vi "DAQmx_Express_mod.vi"(2 "rate":dbl=0.3, 3 "number of samples":i32=1, 4 "timeout (s)":dbl=10.0 format="%0.2f", 5 "error in":errorcluster, 7 "stop (F)":bool, 10 "device name":tag="cDAQ1Mod4") -> (14 "task out":refnum<k21>, 15 "data":dynamicdata(graph), 18 "stopped":bool, 19 "error out":errorcluster)   [LabVIEW 2018]
doc: "Creates, edits, and runs tasks using NI-DAQmx. Refer to the NI-DAQmx Readme for a complete listing of devices NI-DAQmx supports.\n\nWhen you place this Express VI on the block diagram, the DAQ Assistant launches to create a new task. After you create a task, you can double-click the DAQ Assistant Express VI to edit that task. For continuous measurement or generation, place a while loop around the DAQ Assistant Express VI."
uses:
  <vilib>/DAQmx/read.llb/DAQmx Read (Analog 1D Wfm NChan NSamp).vi
  <vilib>/DAQmx/create/channels.llb/DAQmx Create Channel (TEDS-AI-Current-Basic).vi
  <vilib>/DAQmx/create/channels.llb/DAQmx Create Channel (AI-Current-Basic).vi
  <vilib>/DAQmx/configure/timing.llb/DAQmx Timing (Sample Clock).vi
  <vilib>/DAQmx/miscellaneous.llb/DAQmx Fill In Error Info.vi
  <resource>/objmgr/daqmx.rc
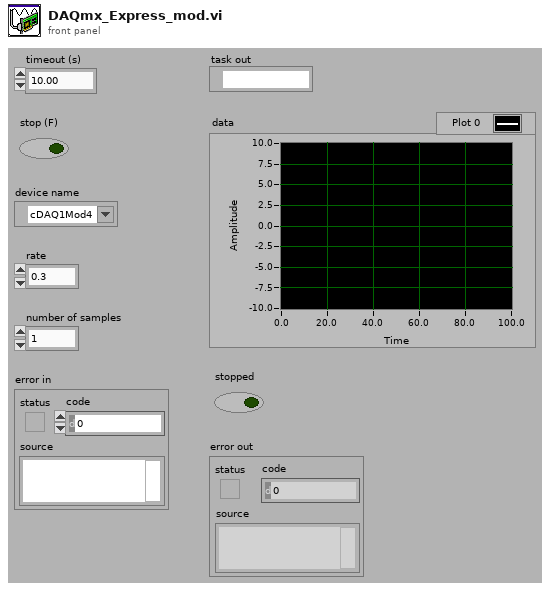
[diagram p1: front panel]
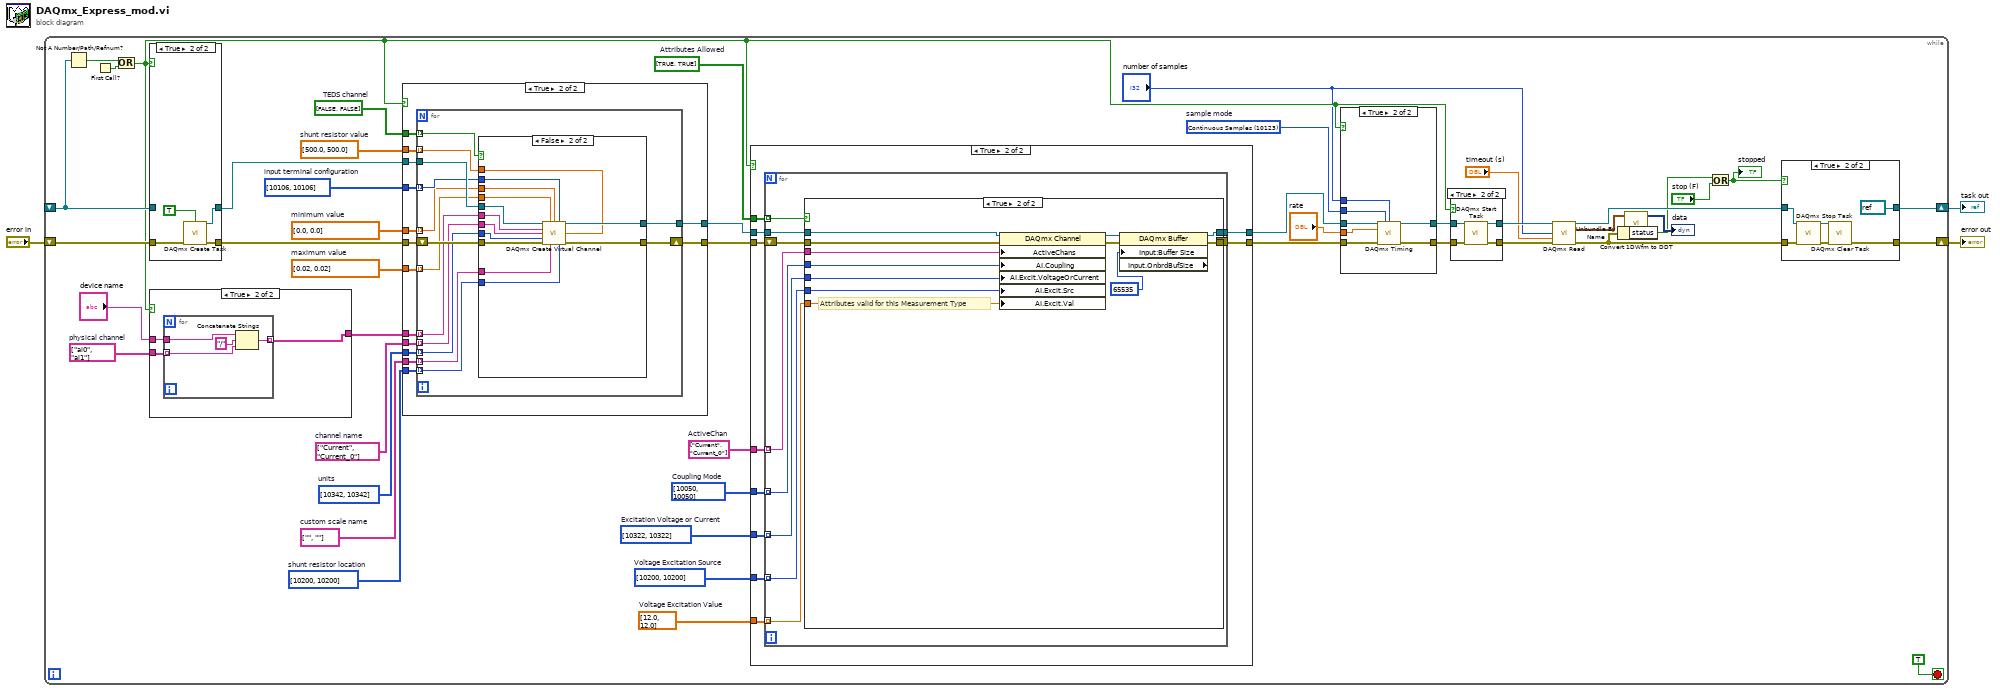
[diagram p0: block diagram]
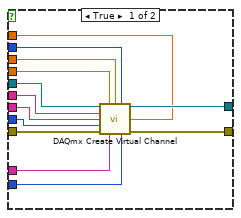
[diagram p8: hidden frame]
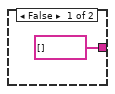
[diagram p9: hidden frame]
diagram:
  n1 = while {
    shift-right: [w10] -> w1
    shift-left: _ -> [w47]
    shift-right: [w8] -> w2
    shift-left: "error in" -> [w48]
    stop <- TRUE stop-if-true
    w20 = 10123 items=["Finite Samples"=10178, "Continuous Samples"=10123, "Hardware Timed Single Point"=12522]  # sample mode
    w24 = bool[] [TRUE, TRUE]  # Attributes Allowed
    w25 = i32[] [10322, 10322] items=["Voltage"=10322, "Current"=10134]  # Excitation Voltage or Current
    w28 = i32[] [10200, 10200] items=["Internal"=10200, "External"=10167, "None"=10230]  # Voltage Excitation Source
    w27 = dbl[] [12.0, 12.0]  # Voltage Excitation Value
    w26 = i32[] [10050, 10050] items=["DC"=10050, "AC"=10045]  # Coupling Mode
    w30 = string[] ["Current", "Current_0"]  # ActiveChan
    w32 = bool[] [FALSE, FALSE]  # TEDS channel
    w34 = i32[] [10200, 10200] items=["Internal"=10200, "External"=10167]  # shunt resistor location
    w33 = dbl[] [500.0, 500.0]  # shunt resistor value
    w35 = string[] ["", ""]  # custom scale name
    w36 = i32[] [10342, 10342] items=["Amps"=10342, "From TEDS"=12516, "From Custom Scale"=10065]  # units
    w37 = string[] ["Current", "Current_0"]  # channel name
    w39 = dbl[] [0.02, 0.02]  # maximum value
    w40 = dbl[] [0.0, 0.0]  # minimum value
    w41 = i32[] [10106, 10106] items=["default"=-1, "RSE"=10083, "NRSE"=10078, "Differential"=10106, "Pseudodifferential"=12529]  # input terminal configuration
    w44 = string[] ["ai0", "ai1"]  # physical channel
    n2 = Not A Number/Path/Refnum?(number/path/refnum=w47) -> (NaN/Path/Refnum?=w46:bool)
    n3 = First Call?() -> (First Call?: T/F=w49:bool)
    n4 = Or(x=w46, y=w49) -> (x .or. y?=w19:bool)
    n5 = case shown="True" w19 {
      tunnel: [w175 w179] -> w43
      tunnel: w47 -> [w175 _]
      tunnel: [w174 w178] -> w42
      tunnel: w48 -> [w174 w176]
      frame False {
      }
      frame True {
        n6 = call <vilib>:"DAQmx Create Task.vi"("auto cleanup"=TRUE, "error in"=w176) -> ("task out"=w179:refnum<k21>, "error out"=w178:errorcluster)  [unwired: 12 in]
      }
    }
    n7 = case shown="True" w19 {
      tunnel: [string[] [] w169] -> w38
      tunnel: "device name" -> [_ w168]
      tunnel: w44 -> [_ w167]
      frame False {
      }
      frame True {
        n8 = for {
          tunnel: [w173] -> w169 mode=indexing
          tunnel: w168 -> [w172]
          tunnel: w167 -> [w170] mode=indexing
          n9 = Concatenate Strings(w172, "/" ("string"), w170) -> (w173:string)
        }
      }
    }
    n10 = case shown="True" w19 {
      tunnel: [w111 w123] -> w29
      tunnel: w43 -> [w111 w125]
      tunnel: [w110 w122] -> w31
      tunnel: w42 -> [w110 w124]
      tunnel: w41 -> [_ w121]
      tunnel: w40 -> [_ w120]
      tunnel: w39 -> [_ w119]
      tunnel: w38 -> [_ w118]
      tunnel: w37 -> [_ w117]
      tunnel: w36 -> [_ w116]
      tunnel: w35 -> [_ w115]
      tunnel: w34 -> [_ w114]
      tunnel: w33 -> [_ w113]
      tunnel: w32 -> [_ w112]
      frame False {
      }
      frame True {
        n11 = for {
          tunnel: w125 -> [w139]
          tunnel: [w137] -> w123
          tunnel: w121 -> [w135] mode=indexing
          tunnel: w120 -> [w134] mode=indexing
          tunnel: w119 -> [w133] mode=indexing
          tunnel: w118 -> [w132] mode=indexing
          tunnel: w117 -> [w131] mode=indexing
          tunnel: w116 -> [w130] mode=indexing
          tunnel: w115 -> [w129] mode=indexing
          shift-right: [w136] -> w122
          shift-left: w124 -> [w138]
          tunnel: w114 -> [w128] mode=indexing
          tunnel: w113 -> [w127] mode=indexing
          tunnel: w112 -> [w126] mode=indexing
          n12 = case shown="False" w126 {
            tunnel: w139 -> [w152 w165]
            tunnel: w138 -> [w151 w164]
            tunnel: [w150 w163] -> w137
            tunnel: [w149 w162] -> w136
            tunnel: w135 -> [w148 w161]
            tunnel: w134 -> [w147 w160]
            tunnel: w133 -> [w146 w159]
            tunnel: w132 -> [w145 w158]
            tunnel: w131 -> [w144 w157]
            tunnel: w130 -> [w143 w156]
            tunnel: w129 -> [w142 w155]
            tunnel: w128 -> [w141 w154]
            tunnel: w127 -> [w140 w153]
            frame True {
              n13 = call-poly <vilib>:"DAQmx Create Virtual Channel.vi"("task in"=w152, "maximum value"=w146, "minimum value"=w147, "input terminal configuration"=w148, "physical channels"=w145, "name to assign"=w144, "external shunt resistor value"=w140, "units"=w143, "error in"=w151, "custom scale name"=w142, "shunt resistor location"=w141) -> ("task out"=w150:refnum<k21>, "error out"=w149:errorcluster)  [unwired: 3 in]
            }
            frame False {
              n14 = call-poly <vilib>:"DAQmx Create Virtual Channel.vi"("task in"=w165, "maximum value"=w159, "minimum value"=w160, "input terminal configuration"=w161, "physical channels"=w158, "name to assign"=w157, "external shunt resistor value"=w153, "units"=w156, "error in"=w164, "custom scale name"=w155, "shunt resistor location"=w154) -> ("task out"=w163:refnum<k21>, "error out"=w162:errorcluster)  [unwired: 3 in]
            }
          }
        }
      }
    }
    n15 = case shown="True" w19 {
      tunnel: [w75 w81] -> w23
      tunnel: w29 -> [w75 w85]
      tunnel: [w74 w83] -> w22
      tunnel: w31 -> [w74 w84]
      tunnel: w30 -> [_ w82]
      tunnel: w28 -> [_ w80]
      tunnel: w27 -> [_ w79]
      tunnel: w26 -> [_ w78]
      tunnel: w25 -> [_ w77]
      tunnel: w24 -> [_ w76]
      frame False {
      }
      frame True {
        n16 = for {
          tunnel: w85 -> [w95]
          shift-right: [w92] -> w83
          shift-left: w84 -> [w93]
          tunnel: w82 -> [w91] mode=indexing
          tunnel: [w94] -> w81
          tunnel: w80 -> [w88] mode=indexing
          tunnel: w79 -> [w89] mode=indexing
          tunnel: w78 -> [w90] mode=indexing
          tunnel: w77 -> [w87] mode=indexing
          tunnel: w76 -> [w86] mode=indexing
          n17 = case shown="True" w86 {
            tunnel: w95 -> [w97 w109]
            tunnel: [w97 w100] -> w94
            tunnel: w93 -> [w96 w108]
            tunnel: [w96 w99] -> w92
            tunnel: w91 -> [_ w107]
            tunnel: w90 -> [_ w106]
            tunnel: w89 -> [_ w105]
            tunnel: w88 -> [_ w104]
            tunnel: w87 -> [_ w103]
            frame False {
              # "Attributes invalid for this Measurement Type"
            }
            frame True {
              # "Attributes valid for this Measurement Type"
              n18 = property class="DAQmx Channel"(reference=w109, error in=w108, "ActiveChans"=w107, "AI.Coupling"=w106, "AI.Excit.VoltageOrCurrent"=w103, "AI.Excit.Src"=w104, "AI.Excit.Val"=w105) -> (reference out=w101:refnum<k21>, error out=w102:errorcluster)
              n19 = property class="DAQmx Buffer" props=["Input:Buffer Size", "Input.OnbrdBufSize"](reference=w101, error in=w102, "Input:Buffer Size"=u16 65535) -> (reference out=w100:refnum<k21>, error out=w99:errorcluster)  [unwired: 1 out]
            }
          }
        }
      }
    }
    n20 = case shown="True" w19 {
      tunnel: [w66 w68] -> w18
      tunnel: w23 -> [w66 w71]
      tunnel: [w65 w67] -> w17
      tunnel: w22 -> [w65 w69]
      tunnel: "number of samples" -> [_ w73]
      tunnel: w20 -> [_ w72]
      tunnel: "rate" -> [_ w70]
      frame False {
      }
      frame True {
        n21 = call-poly <vilib>:"DAQmx Timing.vi"("task/channels in"=w71, "sample mode"=w72, "samples per channel"=w73, "rate"=w70, "error in"=w69) -> ("task out"=w68:refnum<k21>, "error out"=w67:errorcluster)  [unwired: 9 in]
      }
    }
    n22 = case shown="True" w19 {
      tunnel: [w60 w63] -> w16
      tunnel: w18 -> [w60 w64]
      tunnel: [w59 w61] -> w15
      tunnel: w17 -> [w59 w62]
      frame False {
      }
      frame True {
        n23 = call <vilib>:"DAQmx Start Task.vi"("task/channels in"=w64, "error in"=w62) -> ("task out"=w63:refnum<k21>, "error out"=w61:errorcluster)  [unwired: 12 in]
      }
    }
    n24 = call-poly <vilib>:"DAQmx Read.vi"("task/channels in"=w16, "number of samples per channel"="number of samples", "timeout"="timeout (s)", "error in"=w15) -> ("task out"=w9:refnum<k21>, "data"=w13:waveform(dbl)[], "error out"=w7:errorcluster)  [unwired: 9 in]
    n25 = Unbundle By Name(w7) -> ("status"=w6:bool)
    n26 = call <vilib>:"Convert 1DWfm to DDT.vi"("Array of Waveforms"=w13) -> ("Dynamic Data Type"=→"data":dynamicdata)  [unwired: 3 in]
    n27 = Or(x=w6, y="stop (F)") -> (x .or. y?=w4:bool)
    "stopped" <- w4
    n28 = case shown="True" w4 {
      tunnel: [w52 refnum<k21> refnum ("task in")] -> w10
      tunnel: w9 -> [w52 w58]
      tunnel: [w51 w55] -> w8
      tunnel: w7 -> [w51 w57]
      frame False {
      }
      frame True {
        n29 = call <vilib>:"DAQmx Stop Task.vi"("task/channels in"=w58, "error in"=w57) -> ("task out"=w54:refnum<k21>, "error out"=w56:errorcluster)  [unwired: 12 in]
        n30 = call <vilib>:"DAQmx Clear Task.vi"("task in"=w54, "error in"=w56) -> ("error out"=w55:errorcluster)  [unwired: 13 in]
      }
    }
  }
  "error out" <- w2
  "task out" <- w1
